vi "phase_two.vi"() -> ()   [LabVIEW 2015]
uses:
  <vilib>/NXT/Block Support/NXT_OutputPort.ctl
  <vilib>/NXT/Block Support/NXT_InputPort.ctl
  <vilib>/NXT/NXTIO Xnodes/NXTIONodeSubVIs/NXTMotorRunDistance.vi
  <vilib>/NXT/Dual Mode Library/Sensors/EV3_Touch_Reset.vi
  <vilib>/NXT/Dual Mode Library/Sound/Tone.vi
  <vilib>/NXT/Dual Mode Library/Waits/Wait_Num.vi
  <vilib>/NXT/Dual Mode Library/Sensors/Touch_Pressed.vi
  <vilib>/NXT/Dual Mode Library/Waits/Wait_Touch.vi
  <vilib>/NXT/Dual Mode Library/Sensors/EV3_Color_RGB.vi
  global1.vi
  all_done?.vi
  <vilib>/NXT/Subs/LVHSConnector.ctl
  <vilib>/NXT/NXTIO Xnodes/AddressXNode/NXTIOAddress.xnode
  <vilib>/NXT/NXTIO Xnodes/NXTIOXNode/NXTIO.xnode
  <vilib>/NXT/LegoClasses/BrickReference/BrickReference.lvclass
panel:
  in  "Slot 8: Small":dbl=69.0
  in  "Slot 8: Big":dbl=64.0
  in  "Slot 7: Small":dbl=61.0
  in  "Slot 7: Big":dbl=58.0
  in  "Slot 6: Small":dbl=54.0
  in  "Slot 6: Big":dbl=54.0
  in  "Slot 5: Small":dbl=46.0
  in  "Slot 5: Big":dbl=46.0
  in  "Slot 4: Small":dbl=38.0
  in  "Slot 4: Big":dbl=38.0
  in  "Slot 3: Small":dbl=30.0
  in  "Slot 3: Big":dbl=30.0
  in  "Slot 2: Small":dbl=22.0
  in  "Slot 2: Big 3":dbl=22.0
  in  "Slot 1: Small":dbl=16.0
  in  "Slot 1: Big":u32=15
  out "Slot 8: Small":bool
  out "Slot 5: Small":bool
  out "Slot 4: Small":bool
  out "Slot 7: Small":bool
  out "Slot 6: Small":bool
  out "Slot 3: Small":bool
  out "Slot 2: Small":bool
  out "Slot 1: Small":bool
  out "Slot 8: Big":bool
  out "Slot 3: Big":bool
  out "Slot 6: Big":bool
  out "Slot 5: Big":bool
  out "Slot 4: Big":bool
  out "Slot 7: Big":bool
  out "Slot 2: Big":bool
  out "Slot 1: Big":bool
  out "Sum Left":i32
  out "ALL DONE?":bool
  out "Trash/Want Case #":u32
  out "Trash?":bool
  out "4: Type 2 #":u8
  out "3: Type 2 #":u8
  out "2: Type 2 #":u8
  out "1: Type 2 #":u8
  out "4: Type 1 #":u8
  out "3: Type 1 #":u8
  out "2: Type 1 #":u8
  out "1: Type 1 #":u8
  out "4: Compound 2":string
  out "4: Compound 1":string
  out "3: Compound 2":string
  out "3: Compound 1":string
  out "2: Compound 2":string
  out "2: Compound 1":string
  out "1: Compound 2":string
  out "1: Compound 1":string
  out "Full?":bool
  out "Stop?":bool
  out "Current Compound":string
  out "Boolean":bool[](array[boolean])
  in  "B Lower 16":u8
  in  "B Upper 16":u8
  in  "G Lower 16":u8
  in  "G Upper 16":u8
  in  "R Lower 16":u8
  in  "R Upper 16":u8
  in  "B Lower 15":u8
  in  "B Upper 15":u8
  in  "G Lower 15":u8
  in  "G Upper 15":u8
  in  "R Lower 15":u8
  in  "R Upper 15":u8
  in  "B Lower 14":u8
  in  "B Upper 14":u8
  in  "G Lower 14":u8
  in  "G Upper 14":u8
  in  "R Lower 14":u8
  in  "R Upper 14":u8
  in  "B Lower 13":u8
  in  "B Upper 13":u8
  in  "G Lower 13":u8
  in  "G Upper 13":u8
  in  "R Lower 13":u8
  in  "R Upper 13":u8
  in  "B Lower 12":u8=5
  in  "B Upper 12":u8=15
  in  "G Lower 12":u8=77
  in  "G Upper 12":u8=90
  in  "R Lower 12":u8=100
  in  "R Upper 12":u8=130
  in  "B Lower 11":u8=18
  in  "B Upper 11":u8=30
  in  "G Lower 11":u8=120
  in  "G Upper 11":u8=150
  in  "R Lower 11":u8=230
  in  "R Upper 11":u8=255
  in  "B Lower 10":u8=10
  in  "B Upper 10":u8=25
  in  "G Lower 10":u8=10
  in  "G Upper 10":u8=20
  in  "R Lower 10":u8=5
  in  "R Upper 10":u8=15
  in  "B Lower 9":u8=55
  in  "B Upper 9":u8=70
  in  "G Lower 9":u8=20
  in  "G Upper 9":u8=35
  in  "R Lower 9":u8=10
  in  "R Upper 9":u8=20
  out "Bool Number":u32
  in  "B Lower 8":u8=5
  in  "B Upper 8":u8=15
  in  "G Lower 8":u8=15
  in  "G Upper 8":u8=25
  in  "R Lower 8":u8=15
  in  "R Upper 8":u8=30
  in  "B Lower 7":u8=16
  in  "B Upper 7":u8=34
  in  "G Lower 7":u8=40
  in  "G Upper 7":u8=66
  in  "R Lower 7":u8=30
  in  "R Upper 7":u8=55
  in  "B Lower 6":u8=50
  in  "B Upper 6":u8=28
  in  "G Lower 6":u8=66
  in  "G Upper 6":u8=96
  in  "R Lower 6":u8=60
  in  "R Upper 6":u8=87
  in  "B Lower 5":u8=86
  in  "B Upper 5":u16=140
  in  "G Lower 5":u8=130
  in  "G Upper 5":u16=170
  in  "R Lower 5":u16=160
  in  "R Upper 5":u16=220
  in  "B Lower 4":u8=7
  in  "B Upper 4":u8=15
  in  "G Lower 4":u8=7
  in  "G Upper 4":u8=11
  in  "R Lower 4":u8=5
  in  "R Upper 4":u8=10
  in  "B Lower 3":u8=45
  in  "B Upper 3":u8=65
  in  "G Lower 3":u8=20
  in  "G Upper 3":u8=45
  in  "R Lower 3":u8=20
  in  "R Upper 3":u8=40
  in  "B Lower 2":u8
  in  "B Upper 2":u8=5
  in  "G Lower 2":u8
  in  "G Upper 2":u8=10
  in  "R Lower 2":u8=30
  in  "R Upper 2":u8=50
  out "What Type?":string
  in  "Cur B":u8=45
  in  "Cur G":u8=75
  in  "\"Cur\" R":u8=70
  out "What Color?":string
  in  "B Lower":u8
  in  "B Upper":u8=10
  in  "G Lower":u8=2
  in  "G Upper":u8=15
  in  "R Upper":u16=110
  in  "R Lower":u8=60
  out "Cur Blue":u8
  out "Cur Green":u8
  out "Cur Red":u8
  out "Current":cluster{"Red":u8, "Green":u8, "Blue":u8}
  # "DEGREES (ENTER POSITIVE NUMBERS)"
  # "REMEMBER BIG NUMBERS ON TOP, SMALL NUMBERS ON BOTTOM"
  # "Red Big"
  # "Red Small"
  # "Blue Big"
  # "Blue Small"
  # "What is needed?"
  # "Possible errors: \nALSO CURRENTLY IN CONTROL MODE\nNOT IN ACTUAL READ COLOR SENSOR MODE\nFOR TESTING PURPOSES*************\n \nwait/time funcitons in loops\n\nNOT ENOUGH SPACE TO SORT? ELONGATE\nDECIDER!!!!!!!"
  # "White Big"
  # "White Small"
  # "HDPE"
  # "Steel"
  # "1) MOTORS: \nA = Top gate\nB = Bottom gate\nC = Scythe\nD = Decider\n\n2) PORTS:\n1) Color\n2) Touch"
  # "Dark Blue Small"
  # "Yellow Small"
  # "Dark Blue Big"
  # "Yellow Big"
  # "Dark Green Big"
  # "Dark Green Small"
  # "Green Big"
  # "Green Small"
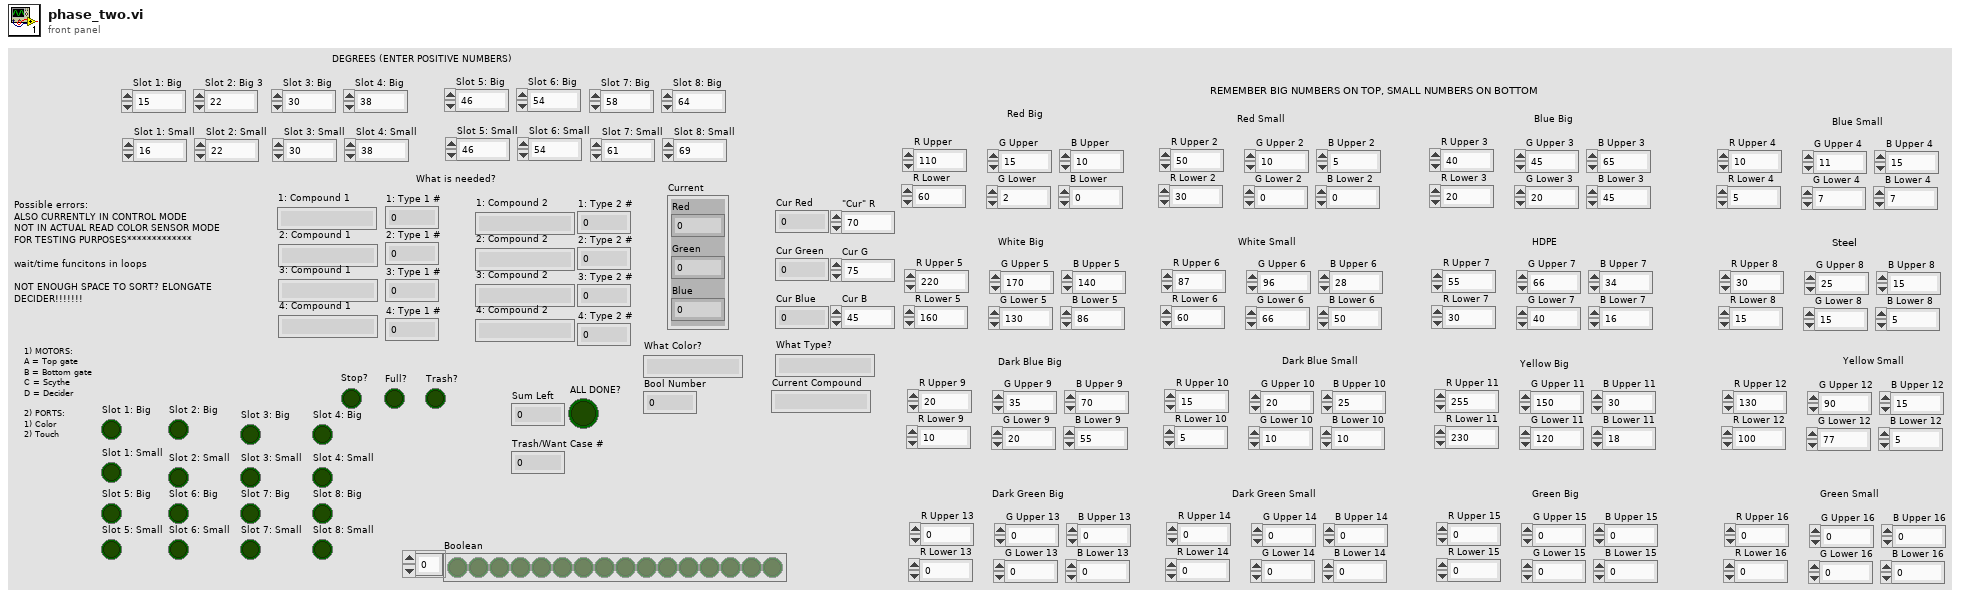
[diagram p1: front panel]
types:
  T1 = typedef "NXT_OutputPort.ctl" = u8
  T2 = typedef "LVHSConnector.ctl" = refnum<class "BrickReference.lvclass">
  T3 = typedef "NXT_InputPort.ctl" = u32
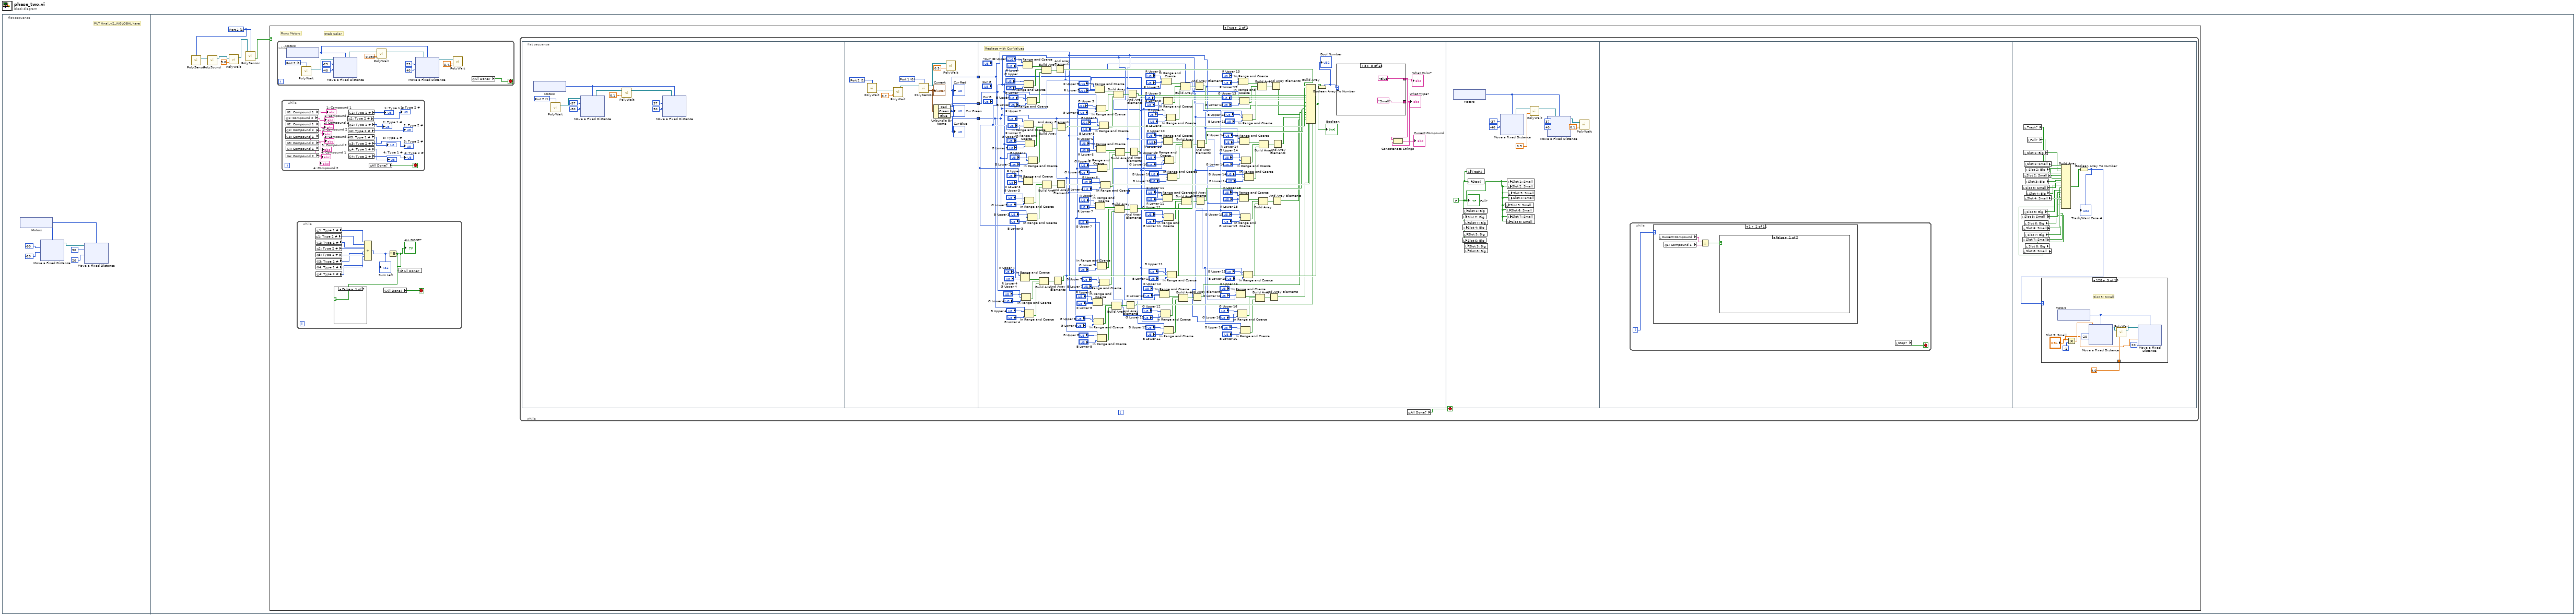
[diagram p0: block diagram]
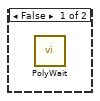
[diagram p2: hidden frame]
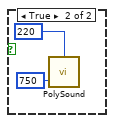
[diagram p3: hidden frame]
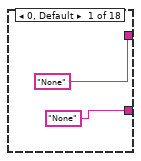
[diagram p4: hidden frame]
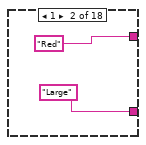
[diagram p5: hidden frame]
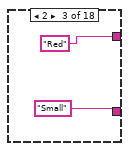
[diagram p6: hidden frame]
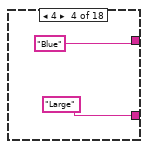
[diagram p7: hidden frame]
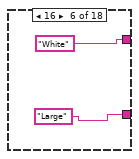
[diagram p8: hidden frame]
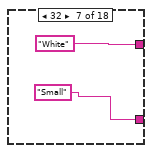
[diagram p9: hidden frame]
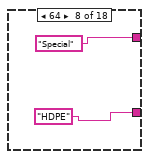
[diagram p10: hidden frame]
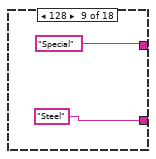
[diagram p11: hidden frame]
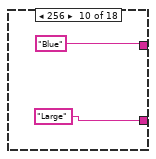
[diagram p12: hidden frame]
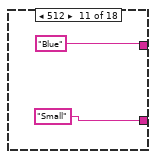
[diagram p13: hidden frame]
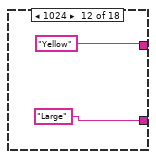
[diagram p14: hidden frame]
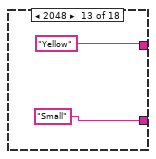
[diagram p15: hidden frame]
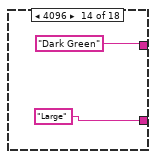
[diagram p16: hidden frame]
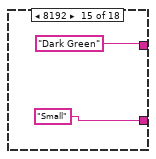
[diagram p17: hidden frame]
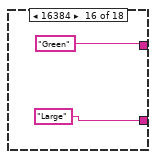
[diagram p18: hidden frame]
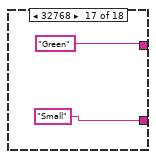
[diagram p19: hidden frame]
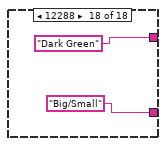
[diagram p20: hidden frame]
diagram:
  n1 = flat-sequence {
    frame #0 {
      # "PUT final_v2_WGLOBAL here"
      n2 = xnode "Motors"() -> ("Motor"=w6:T1)
      n3 = xnode "Move a Fixed Distance"("Speed 1"=-20, "Distance 1"=-90, "Motors"=w6) -> ("NXT/EV3"=w5:T2)  [unwired: 1 in]
      n4 = xnode "Move a Fixed Distance"("Speed 1"=20, "Distance 1"=90, "Motors"=w6, "NXT/EV3"=w5) -> ()  [unwired: 1 out]
    }
    frame #1 {
      w28 = T3 1 items=["Port 1", "Port 2", "Port 3", "Port 4"] ("Port (Port 1)")
      n5 = call-poly <vilib>:"PolySensor.vi"("Port (Port 1)"=w28) -> ("NXT/EV3"=w32:T2)  [unwired: 3 in]
      n6 = call-poly <vilib>:"PolySound.vi"("NXT/EV3"=w32) -> ("NXT/EV3"=w31:T2)  [unwired: 3 in]
      n7 = call-poly <vilib>:"PolyWait.vi"("Time (1 sec)"=sgl 5.0, "NXT/EV3"=w31) -> ("NXT/EV3"=w30:T2)  [unwired: 2 in]
      n8 = call-poly <vilib>:"PolySensor.vi"("NXT/EV3"=w30, "Port (Port 1)"=w28) -> ("Yes / No"=w33:bool)  [unwired: 1 in, 1 out]
      n9 = case shown="True" w33 {
        frame False {
          n10 = call-poly <vilib>:"PolyWait.vi"() -> ()  [unwired: 4 in, 1 out]
        }
        frame True {
          # "Grab Color"
          # "Runs Motors"
          n11 = while {
            stop <- w37 stop-if-true
            w39 = T3 1 items=["Port 1", "Port 2", "Port 3", "Port 4"] ("Port (Port 1)")
            n12 = xnode "Motors"() -> ("Motor"=w45:T1)
            n13 = call-poly <vilib>:"PolyWait.vi"("Port (Port 1)"=w39) -> ("NXT/EV3"=w38:T2)  [unwired: 3 in]
            n14 = xnode "Move a Fixed Distance"("Speed 1"=i8 -40, "Distance 1"=-25, "Motors"=w45, "NXT/EV3"=w38) -> ("NXT/EV3"=w44:T2)
            n15 = call-poly <vilib>:"PolyWait.vi"("Time (1 sec)"=sgl 0.05, "NXT/EV3"=w44) -> ("NXT/EV3"=w43:T2)  [unwired: 2 in]
            n16 = xnode "Move a Fixed Distance"("Speed 1"=i8 40, "Distance 1"=25, "Motors"=w45, "NXT/EV3"=w43) -> ("NXT/EV3"=w34:T2)
            n17 = call-poly <vilib>:"PolyWait.vi"("Time (1 sec)"=sgl 0.4, "NXT/EV3"=w34) -> ()  [unwired: 2 in, 1 out]
            n18 = global read "all_done?.vi" "All Done?"() -> (w37:bool)
          }
          n19 = while {
            stop <- w81 stop-if-true
            n20 = global read "global1.vi" "1: Compound 2"() -> (→"1: Compound 2":string)
            n21 = global read "global1.vi" "2: Compound 2"() -> (→"2: Compound 2":string)
            n22 = global read "global1.vi" "3: Compound 1"() -> (→"3: Compound 1":string)
            n23 = global read "global1.vi" "1: Compound 1"() -> (→"1: Compound 1":string)
            n24 = global read "global1.vi" "2: Compound 1"() -> (→"2: Compound 1":string)
            n25 = global read "global1.vi" "3: Compound 2"() -> (→"3: Compound 2":string)
            n26 = global read "global1.vi" "4: Compound 1"() -> (→"4: Compound 1":string)
            n27 = global read "global1.vi" "4: Compound 2"() -> (→"4: Compound 2":string)
            n28 = global read "global1.vi" "1: Type 2 #"() -> (→"1: Type 2 #":i32)
            n29 = global read "global1.vi" "2: Type 2 #"() -> (→"2: Type 2 #":i32)
            n30 = global read "global1.vi" "3: Type 1 #"() -> (→"3: Type 1 #":i32)
            n31 = global read "global1.vi" "1: Type 1 #"() -> (→"1: Type 1 #":i32)
            n32 = global read "global1.vi" "2: Type 1 #"() -> (→"2: Type 1 #":i32)
            n33 = global read "global1.vi" "3: Type 2 #"() -> (→"3: Type 2 #":i32)
            n34 = global read "global1.vi" "4: Type 1 #"() -> (→"4: Type 1 #":i32)
            n35 = global read "global1.vi" "4: Type 2 #"() -> (→"4: Type 2 #":i32)
            n36 = global read "all_done?.vi" "All Done?"() -> (w81:bool)
          }
          n37 = while {
            stop <- w70 stop-if-true
            n38 = global read "global1.vi" "1: Type 2 #"() -> (w77:i32)
            n39 = global read "global1.vi" "2: Type 2 #"() -> (w75:i32)
            n40 = global read "global1.vi" "3: Type 1 #"() -> (w74:i32)
            n41 = global read "global1.vi" "1: Type 1 #"() -> (w78:i32)
            n42 = global read "global1.vi" "2: Type 1 #"() -> (w76:i32)
            n43 = global read "global1.vi" "3: Type 2 #"() -> (w73:i32)
            n44 = global read "global1.vi" "4: Type 1 #"() -> (w72:i32)
            n45 = global read "global1.vi" "4: Type 2 #"() -> (w71:i32)
            n46 = Compound Arithmetic op=ADD(w78, w77, w76, w75, w74, w73, w72, w71) -> (w69:i32)
            "Sum Left" <- w69
            n47 = global read "all_done?.vi" "All Done?"() -> (w70:bool)
            n48 = Equal To 0?(x=w69) -> (x = 0?=w68:bool)
            "ALL DONE?" <- w68
            n49 = case shown="False" w68 {
              frame False {
              }
              frame True {
                n50 = call-poly <vilib>:"PolySound.vi"("Duration (500 ms)"=u16 750, "Tone (440 Hz)"=u16 220) -> ()  [unwired: 2 in, 1 out]
              }
            }
            n51 = global write "all_done?.vi" "All Done?"(w68) -> ()
          }
          n52 = while {
            stop <- w101 stop-if-true
            n53 = flat-sequence {
              tunnel: [w135] -> w100
              tunnel: [w134] -> w99
              tunnel: [w133] -> w98
              tunnel: w100 -> [w146]
              tunnel: w99 -> [w145]
              tunnel: w98 -> [w144]
              frame #0 {
                w103 = T3 1 items=["Port 1", "Port 2", "Port 3", "Port 4"] ("Port (Port 1)")
                n54 = xnode "Motors"() -> ("Motor"=w110:T1)
                n55 = call-poly <vilib>:"PolyWait.vi"("Port (Port 1)"=w103) -> ("NXT/EV3"=w102:T2)  [unwired: 3 in]
                n56 = xnode "Move a Fixed Distance"("Speed 1"=i8 -50, "Distance 1"=-37, "Motors"=w110, "NXT/EV3"=w102) -> ("NXT/EV3"=w109:T2)
                n57 = call-poly <vilib>:"PolyWait.vi"("Time (1 sec)"=0.1, "NXT/EV3"=w109) -> ("NXT/EV3"=w108:T2)  [unwired: 2 in]
                n58 = xnode "Move a Fixed Distance"("Speed 1"=i8 50, "Distance 1"=37, "Motors"=w110, "NXT/EV3"=w108) -> ()  [unwired: 1 out]
              }
              frame #1 {
                w139 = T3 0 items=["Port 1", "Port 2", "Port 3", "Port 4"] ("Port (Port 1)")
                w142 = T3 1 items=["Port 1", "Port 2", "Port 3", "Port 4"] ("Port (Port 1)")
                n59 = call-poly <vilib>:"PolyWait.vi"("Port (Port 1)"=w142) -> ("NXT/EV3"=w141:T2)  [unwired: 3 in]
                n60 = call-poly <vilib>:"PolyWait.vi"("Time (1 sec)"=0.7, "NXT/EV3"=w141) -> ("NXT/EV3"=w140:T2)  [unwired: 2 in]
                n61 = call-poly <vilib>:"PolySensor.vi"("NXT/EV3"=w140, "Port (Port 1)"=w139) -> ("RGB Color"=w138:cluster{"Red":u8, "Green":u8, "Blue":u8}, "NXT/EV3"=w137:T2)  [unwired: 1 in]
                "Current" <- w138
                n62 = Unbundle By Name(w138) -> ("Red"=w135:u8, "Green"=w134:u8, "Blue"=w133:u8)
                "Cur Green" <- w134
                "Cur Red" <- w135
                "Cur Blue" <- w133
                n63 = call-poly <vilib>:"PolyWait.vi"("Time (1 sec)"=sgl 0.5, "NXT/EV3"=w137) -> ()  [unwired: 2 in, 1 out]
              }
              frame #2 {
                # "Replace with Cur Values"
                n64 = In Range and Coerce(upper limit="R Upper 4", x=w146, lower limit="R Lower 4") -> (In Range?=w288:bool)  [unwired: 1 out]
                n65 = In Range and Coerce(upper limit="G Upper 4", x=w145, lower limit="G Lower 4") -> (In Range?=w287:bool)  [unwired: 1 out]
                n66 = In Range and Coerce(upper limit="R Upper", x=w146, lower limit="R Lower") -> (In Range?=w321:bool)  [unwired: 1 out]
                n67 = In Range and Coerce(upper limit="R Upper 3", x=w146, lower limit="R Lower 3") -> (In Range?=w298:bool)  [unwired: 1 out]
                n68 = In Range and Coerce(upper limit="G Upper", x=w145, lower limit="G Lower") -> (In Range?=w320:bool)  [unwired: 1 out]
                n69 = In Range and Coerce(upper limit="R Upper 2", x=w146, lower limit="R Lower 2") -> (In Range?=w310:bool)  [unwired: 1 out]
                n70 = In Range and Coerce(upper limit="G Upper 3", x=w145, lower limit="G Lower 3") -> (In Range?=w297:bool)  [unwired: 1 out]
                n71 = In Range and Coerce(upper limit="B Upper 4", x=w144, lower limit="B Lower 4") -> (In Range?=w285:bool)  [unwired: 1 out]
                n72 = In Range and Coerce(upper limit="G Upper 2", x=w145, lower limit="G Lower 2") -> (In Range?=w309:bool)  [unwired: 1 out]
                n73 = In Range and Coerce(upper limit="B Upper", x=w144, lower limit="B Lower") -> (In Range?=w306:bool)  [unwired: 1 out]
                n74 = In Range and Coerce(upper limit="B Upper 3", x=w144, lower limit="B Lower 3") -> (In Range?=w295:bool)  [unwired: 1 out]
                n75 = In Range and Coerce(upper limit="B Upper 2", x=w144, lower limit="B Lower 2") -> (In Range?=w305:bool)  [unwired: 1 out]
                n76 = Build Array(w288, w287, w285) -> (w286:bool[])
                n77 = Build Array(w321, w320, w306) -> (w319:bool[])
                n78 = Build Array(w298, w297, w295) -> (w296:bool[])
                n79 = Build Array(w310, w309, w305) -> (w308:bool[])
                n80 = And Array Elements(Boolean array=w286) -> (logical AND=w284:bool)
                n81 = And Array Elements(Boolean array=w319) -> (logical AND=w318:bool)
                n82 = And Array Elements(Boolean array=w296) -> (logical AND=w283:bool)
                n83 = And Array Elements(Boolean array=w308) -> (logical AND=w307:bool)
                n84 = In Range and Coerce(upper limit="R Upper 8", x=w146, lower limit="R Lower 8") -> (In Range?=w246:bool)  [unwired: 1 out]
                n85 = In Range and Coerce(upper limit="G Upper 8", x=w145, lower limit="G Lower 8") -> (In Range?=w245:bool)  [unwired: 1 out]
                n86 = In Range and Coerce(upper limit="R Upper 5", x=w146, lower limit="R Lower 5") -> (In Range?=w276:bool)  [unwired: 1 out]
                n87 = In Range and Coerce(upper limit="R Upper 7", x=w146, lower limit="R Lower 7") -> (In Range?=w256:bool)  [unwired: 1 out]
                n88 = In Range and Coerce(upper limit="G Upper 5", x=w145, lower limit="G Lower 5") -> (In Range?=w275:bool)  [unwired: 1 out]
                n89 = In Range and Coerce(upper limit="R Upper 6", x=w146, lower limit="R Lower 6") -> (In Range?=w267:bool)  [unwired: 1 out]
                n90 = In Range and Coerce(upper limit="G Upper 7", x=w145, lower limit="G Lower 7") -> (In Range?=w255:bool)  [unwired: 1 out]
                n91 = In Range and Coerce(upper limit="B Upper 8", x=w144, lower limit="B Lower 8") -> (In Range?=w243:bool)  [unwired: 1 out]
                n92 = In Range and Coerce(upper limit="G Upper 6", x=w145, lower limit="G Lower 6") -> (In Range?=w266:bool)  [unwired: 1 out]
                n93 = In Range and Coerce(upper limit="B Upper 5", x=w144, lower limit="B Lower 5") -> (In Range?=w264:bool)  [unwired: 1 out]
                n94 = In Range and Coerce(upper limit="B Upper 7", x=w144, lower limit="B Lower 7") -> (In Range?=w253:bool)  [unwired: 1 out]
                n95 = In Range and Coerce(upper limit="B Upper 6", x=w144, lower limit="B Lower 6") -> (In Range?=w263:bool)  [unwired: 1 out]
                n96 = Build Array(w246, w245, w243) -> (w244:bool[])
                n97 = Build Array(w276, w275, w264) -> (w274:bool[])
                n98 = Build Array(w256, w255, w253) -> (w254:bool[])
                n99 = Build Array(w267, w266, w263) -> (w265:bool[])
                n100 = And Array Elements(Boolean array=w244) -> (logical AND=w239:bool)
                n101 = And Array Elements(Boolean array=w274) -> (logical AND=w242:bool)
                n102 = And Array Elements(Boolean array=w254) -> (logical AND=w240:bool)
                n103 = And Array Elements(Boolean array=w265) -> (logical AND=w241:bool)
                n104 = In Range and Coerce(upper limit="R Upper 12", x=w146, lower limit="R Lower 12") -> (In Range?=w201:bool)  [unwired: 1 out]
                n105 = In Range and Coerce(upper limit="G Upper 12", x=w145, lower limit="G Lower 12") -> (In Range?=w200:bool)  [unwired: 1 out]
                n106 = In Range and Coerce(upper limit="R Upper 9", x=w146, lower limit="R Lower 9") -> (In Range?=w231:bool)  [unwired: 1 out]
                n107 = In Range and Coerce(upper limit="R Upper 11", x=w146, lower limit="R Lower 11") -> (In Range?=w211:bool)  [unwired: 1 out]
                n108 = In Range and Coerce(upper limit="G Upper 9", x=w145, lower limit="G Lower 9") -> (In Range?=w230:bool)  [unwired: 1 out]
                n109 = In Range and Coerce(upper limit="R Upper 10", x=w146, lower limit="R Lower 10") -> (In Range?=w222:bool)  [unwired: 1 out]
                n110 = In Range and Coerce(upper limit="G Upper 11", x=w145, lower limit="G Lower 11") -> (In Range?=w210:bool)  [unwired: 1 out]
                n111 = In Range and Coerce(upper limit="B Upper 12", x=w144, lower limit="B Lower 12") -> (In Range?=w198:bool)  [unwired: 1 out]
                n112 = In Range and Coerce(upper limit="G Upper 10", x=w145, lower limit="G Lower 10") -> (In Range?=w221:bool)  [unwired: 1 out]
                n113 = In Range and Coerce(upper limit="B Upper 9", x=w144, lower limit="B Lower 9") -> (In Range?=w219:bool)  [unwired: 1 out]
                n114 = In Range and Coerce(upper limit="B Upper 11", x=w144, lower limit="B Lower 11") -> (In Range?=w208:bool)  [unwired: 1 out]
                n115 = In Range and Coerce(upper limit="B Upper 10", x=w144, lower limit="B Lower 10") -> (In Range?=w218:bool)  [unwired: 1 out]
                n116 = Build Array(w201, w200, w198) -> (w199:bool[])
                n117 = Build Array(w231, w230, w219) -> (w229:bool[])
                n118 = Build Array(w211, w210, w208) -> (w209:bool[])
                n119 = Build Array(w222, w221, w218) -> (w220:bool[])
                n120 = And Array Elements(Boolean array=w199) -> (logical AND=w154:bool)
                n121 = And Array Elements(Boolean array=w229) -> (logical AND=w157:bool)
                n122 = And Array Elements(Boolean array=w209) -> (logical AND=w155:bool)
                n123 = And Array Elements(Boolean array=w220) -> (logical AND=w156:bool)
                n124 = In Range and Coerce(upper limit="R Upper 16", x=w146, lower limit="R Lower 16") -> (In Range?=w161:bool)  [unwired: 1 out]
                n125 = In Range and Coerce(upper limit="G Upper 16", x=w145, lower limit="G Lower 16") -> (In Range?=w160:bool)  [unwired: 1 out]
                n126 = In Range and Coerce(upper limit="R Upper 13", x=w146, lower limit="R Lower 13") -> (In Range?=w191:bool)  [unwired: 1 out]
                n127 = In Range and Coerce(upper limit="R Upper 15", x=w146, lower limit="R Lower 15") -> (In Range?=w171:bool)  [unwired: 1 out]
                n128 = In Range and Coerce(upper limit="G Upper 13", x=w145, lower limit="G Lower 13") -> (In Range?=w190:bool)  [unwired: 1 out]
                n129 = In Range and Coerce(upper limit="R Upper 14", x=w146, lower limit="R Lower 14") -> (In Range?=w182:bool)  [unwired: 1 out]
                n130 = In Range and Coerce(upper limit="G Upper 15", x=w145, lower limit="G Lower 15") -> (In Range?=w170:bool)  [unwired: 1 out]
                n131 = In Range and Coerce(upper limit="B Upper 16", x=w144, lower limit="B Lower 16") -> (In Range?=w158:bool)  [unwired: 1 out]
                n132 = In Range and Coerce(upper limit="G Upper 14", x=w145, lower limit="G Lower 14") -> (In Range?=w181:bool)  [unwired: 1 out]
                n133 = In Range and Coerce(upper limit="B Upper 13", x=w144, lower limit="B Lower 13") -> (In Range?=w179:bool)  [unwired: 1 out]
                n134 = In Range and Coerce(upper limit="B Upper 15", x=w144, lower limit="B Lower 15") -> (In Range?=w168:bool)  [unwired: 1 out]
                n135 = In Range and Coerce(upper limit="B Upper 14", x=w144, lower limit="B Lower 14") -> (In Range?=w178:bool)  [unwired: 1 out]
                n136 = Build Array(w161, w160, w158) -> (w159:bool[])
                n137 = Build Array(w191, w190, w179) -> (w189:bool[])
                n138 = Build Array(w171, w170, w168) -> (w169:bool[])
                n139 = Build Array(w182, w181, w178) -> (w180:bool[])
                n140 = And Array Elements(Boolean array=w159) -> (logical AND=w150:bool)
                n141 = And Array Elements(Boolean array=w189) -> (logical AND=w153:bool)
                n142 = And Array Elements(Boolean array=w169) -> (logical AND=w151:bool)
                n143 = And Array Elements(Boolean array=w180) -> (logical AND=w152:bool)
                n144 = Build Array(w318, w307, w283, w284, w242, w241, w240, w239, w157, w156, w155, w154, w153, w152, w151, w150) -> (w317:bool[])
                "Boolean" <- w317
                n145 = Boolean Array To Number(Boolean array=w317) -> (number=w238:u32)
                "Bool Number" <- w238
                n146 = case shown="8" w238 {
                  tunnel: ["None" "Red" "Red" "Blue" "Blue" "White" "White" "Special" "Special" "Blue" "Blue" "Yellow" "Yellow" "Dark Green" "Dark Green" "Green" "Green" "Dark Green"] -> w149
                  tunnel: ["None" "Large" "Small" "Large" "Small" "Large" "Small" "HDPE" "Steel" "Large" "Small" "Large" "Small" "Large" "Small" "Large" "Small" "Big/Small"] -> w148
                  frame 0, Default {
                  }
                  frame 1 {
                  }
                  frame 2 {
                  }
                  frame 4 {
                  }
                  frame 8 {
                  }
                  frame 16 {
                  }
                  frame 32 {
                  }
                  frame 64 {
                  }
                  frame 128 {
                  }
                  frame 256 {
                  }
                  frame 512 {
                  }
                  frame 1024 {
                  }
                  frame 2048 {
                  }
                  frame 4096 {
                  }
                  frame 8192 {
                  }
                  frame 16384 {
                  }
                  frame 32768 {
                  }
                  frame 12288 {
                  }
                }
                "What Color?" <- w149
                "What Type?" <- w148
                n147 = Concatenate Strings(w149, w148) -> (→"Current Compound":string)
              }
              frame #3 {
                w366 = FALSE
                n148 = xnode "Motors"() -> ("Motor"=w372:T1)
                n149 = local write "Slot 2: Big"(w366) -> ()
                n150 = local write "Slot 6: Big"(w366) -> ()
                n151 = local write "Slot 4: Big"(w366) -> ()
                n152 = local write "Slot 1: Big"(w366) -> ()
                n153 = local write "Slot 5: Big"(w366) -> ()
                n154 = local write "Slot 7: Big"(w366) -> ()
                n155 = local write "Slot 3: Big"(w366) -> ()
                n156 = local write "Slot 8: Big"(w366) -> ()
                n157 = local write "Trash?"(w366) -> ()
                n158 = local write "Stop?"(w366) -> ()
                n159 = xnode "Move a Fixed Distance"("Speed 1"=i8 -40 ("Power/Speed 1"), "Distance 1"=-37, "Motors"=w372) -> ("NXT/EV3"=w374:T2)  [unwired: 1 in]
                n160 = local write "Slot 5: Small"(w366) -> ()
                n161 = local write "Slot 6: Small"(w366) -> ()
                n162 = local write "Slot 8: Small"(w366) -> ()
                n163 = local write "Slot 1: Small"(w366) -> ()
                n164 = local write "Slot 2: Small"(w366) -> ()
                n165 = local write "Slot 7: Small"(w366) -> ()
                n166 = local write "Slot 3: Small"(w366) -> ()
                n167 = local write "Slot 4: Small"(w366) -> ()
                n168 = call-poly <vilib>:"PolyWait.vi"("Time (1 sec)"=0.3, "NXT/EV3"=w374) -> ("NXT/EV3"=w373:T2)  [unwired: 2 in]
                n169 = xnode "Move a Fixed Distance"("Speed 1"=i8 40, "Distance 1"=37, "Motors"=w372, "NXT/EV3"=w373) -> ("NXT/EV3"=w364:T2)
                n170 = call-poly <vilib>:"PolyWait.vi"("Time (1 sec)"=sgl 0.1, "NXT/EV3"=w364) -> ()  [unwired: 2 in, 1 out]
                "Full?" <- w366
              }
              frame #4 {
                n171 = while {
                  i -> [w396]
                  stop <- w397 stop-if-true
                  n172 = case shown="1" w396 {
                    frame 0, Default {
                    }
                    frame 1 {
                      n173 = local read "Current Compound"() -> (w400:string)
                      n174 = global read "global1.vi" "1: Compound 1"() -> (w399:string)
                      n175 = Equal?(x=w400, y=w399) -> (x = y?=w398:bool)
                      n176 = case shown="False" w398 {
                        frame False {
                        }
                        frame True {
                          n177 = global read "global1.vi" "1: Type 1 #"() -> (w402:i32)
                          n178 = Greater?(x=w402, y=u32 0) -> (0:w401:bool)
                          n179 = case shown="False" w401 {
                            frame False {
                              n180 = local write "Stop?"(TRUE) -> ()
                              "Slot 5: Big" <- TRUE
                            }
                            frame True {
                              n181 = global read "global1.vi" "1: Type 1 #"() -> (w409:i32)
                              n182 = Decrement(x=w409) -> (x-1=w408:i32)
                              n183 = global write "global1.vi" "1: Type 1 #"(w408) -> ()
                              "Stop?" <- TRUE
                              "Slot 1: Big" <- TRUE
                            }
                          }
                        }
                      }
                    }
                    frame 2 {
                      n184 = local read "Current Compound"() -> (w412:string)
                      n185 = global read "global1.vi" "1: Compound 2"() -> (w411:string)
                      n186 = Equal?(x=w412, y=w411) -> (x = y?=w410:bool)
                      n187 = case shown="True" w410 {
                        frame False {
                        }
                        frame True {
                          n188 = global read "global1.vi" "1: Type 2 #"() -> (w414:i32)
                          n189 = Greater?(x=w414, y=u32 0) -> (0:w413:bool)
                          n190 = case shown="False" w413 {
                            frame False {
                              n191 = local write "Stop?"(TRUE) -> ()
                              "Slot 5: Small" <- TRUE
                            }
                            frame True {
                              n192 = global read "global1.vi" "1: Type 2 #"() -> (w421:i32)
                              n193 = local write "Stop?"(TRUE) -> ()
                              n194 = Decrement(x=w421) -> (x-1=w420:i32)
                              n195 = global write "global1.vi" "1: Type 2 #"(w420) -> ()
                              "Slot 1: Small" <- TRUE
                            }
                          }
                        }
                      }
                    }
                    frame 3 {
                      n196 = local read "Current Compound"() -> (w424:string)
                      n197 = global read "global1.vi" "2: Compound 1"() -> (w423:string)
                      n198 = Equal?(x=w424, y=w423) -> (x = y?=w422:bool)
                      n199 = case shown="True" w422 {
                        frame False {
                        }
                        frame True {
                          n200 = global read "global1.vi" "2: Type 1 #"() -> (w426:i32)
                          n201 = Greater?(x=w426, y=u32 0) -> (0:w425:bool)
                          n202 = case shown="True" w425 {
                            frame False {
                              n203 = local write "Stop?"(TRUE) -> ()
                              "Slot 6: Big" <- TRUE
                            }
                            frame True {
                              n204 = global read "global1.vi" "2: Type 1 #"() -> (w433:i32)
                              n205 = local write "Stop?"(TRUE) -> ()
                              n206 = Decrement(x=w433) -> (x-1=w432:i32)
                              n207 = global write "global1.vi" "2: Type 1 #"(w432) -> ()
                              "Slot 2: Big" <- TRUE
                            }
                          }
                        }
                      }
                    }
                    frame 4 {
                      n208 = local read "Current Compound"() -> (w436:string)
                      n209 = global read "global1.vi" "2: Compound 2"() -> (w435:string)
                      n210 = Equal?(x=w436, y=w435) -> (x = y?=w434:bool)
                      n211 = case shown="True" w434 {
                        frame False {
                        }
                        frame True {
                          n212 = global read "global1.vi" "2: Type 2 #"() -> (w438:i32)
                          n213 = Greater?(x=w438, y=u32 0) -> (0:w437:bool)
                          n214 = case shown="False" w437 {
                            frame False {
                              n215 = local write "Stop?"(TRUE) -> ()
                              "Slot 6: Small" <- TRUE
                            }
                            frame True {
                              n216 = global read "global1.vi" "2: Type 2 #"() -> (w445:i32)
                              n217 = local write "Stop?"(TRUE) -> ()
                              n218 = Decrement(x=w445) -> (x-1=w444:i32)
                              n219 = global write "global1.vi" "2: Type 2 #"(w444) -> ()
                              "Slot 2: Small" <- TRUE
                            }
                          }
                        }
                      }
                    }
                    frame 5 {
                      n220 = local read "Current Compound"() -> (w448:string)
                      n221 = global read "global1.vi" "3: Compound 1"() -> (w447:string)
                      n222 = Equal?(x=w448, y=w447) -> (x = y?=w446:bool)
                      n223 = case shown="True" w446 {
                        frame False {
                        }
                        frame True {
                          n224 = global read "global1.vi" "3: Type 1 #"() -> (w450:i32)
                          n225 = Greater?(x=w450, y=u32 0) -> (0:w449:bool)
                          n226 = case shown="True" w449 {
                            frame False {
                              n227 = local write "Stop?"(TRUE) -> ()
                              "Slot 3: Big" <- TRUE
                            }
                            frame True {
                              n228 = global read "global1.vi" "3: Type 1 #"() -> (w457:i32)
                              n229 = local write "Stop?"(TRUE) -> ()
                              n230 = Decrement(x=w457) -> (x-1=w456:i32)
                              n231 = global write "global1.vi" "3: Type 1 #"(w456) -> ()
                              "Slot 7: Big" <- TRUE
                            }
                          }
                        }
                      }
                    }
                    frame 6 {
                      n232 = local read "Current Compound"() -> (w460:string)
                      n233 = global read "global1.vi" "3: Compound 2"() -> (w459:string)
                      n234 = Equal?(x=w460, y=w459) -> (x = y?=w458:bool)
                      n235 = case shown="True" w458 {
                        frame False {
                        }
                        frame True {
                          n236 = global read "global1.vi" "3: Type 2 #"() -> (w462:i32)
                          n237 = Greater?(x=w462, y=u32 0) -> (0:w461:bool)
                          n238 = case shown="False" w461 {
                            frame False {
                              n239 = local write "Stop?"(TRUE) -> ()
                              "Slot 7: Small" <- TRUE
                            }
                            frame True {
                              n240 = global read "global1.vi" "3: Type 2 #"() -> (w469:i32)
                              n241 = local write "Stop?"(TRUE) -> ()
                              n242 = Decrement(x=w469) -> (x-1=w468:i32)
                              n243 = global write "global1.vi" "3: Type 2 #"(w468) -> ()
                              "Slot 3: Small" <- TRUE
                            }
                          }
                        }
                      }
                    }
                    frame 7 {
                      n244 = local read "Current Compound"() -> (w472:string)
                      n245 = global read "global1.vi" "4: Compound 1"() -> (w471:string)
                      n246 = Equal?(x=w472, y=w471) -> (x = y?=w470:bool)
                      n247 = case shown="True" w470 {
                        frame False {
                        }
                        frame True {
                          n248 = global read "global1.vi" "4: Type 1 #"() -> (w474:i32)
                          n249 = Greater?(x=w474, y=u32 0) -> (0:w473:bool)
                          n250 = case shown="False" w473 {
                            frame False {
                              n251 = local write "Stop?"(TRUE) -> ()
                              "Slot 8: Big" <- TRUE
                            }
                            frame True {
                              n252 = global read "global1.vi" "4: Type 1 #"() -> (w481:i32)
                              n253 = local write "Stop?"(TRUE) -> ()
                              n254 = Decrement(x=w481) -> (x-1=w480:i32)
                              n255 = global write "global1.vi" "4: Type 1 #"(w480) -> ()
                              "Slot 4: Big" <- TRUE
                            }
                          }
                        }
                      }
                    }
                    frame 8 {
                      n256 = local read "Current Compound"() -> (w484:string)
                      n257 = global read "global1.vi" "4: Compound 2"() -> (w483:string)
                      n258 = Equal?(x=w484, y=w483) -> (x = y?=w482:bool)
                      n259 = case shown="True" w482 {
                        frame False {
                        }
                        frame True {
                          n260 = global read "global1.vi" "4: Type 2 #"() -> (w486:i32)
                          n261 = Greater?(x=w486, y=u32 0) -> (0:w485:bool)
                          n262 = case shown="False" w485 {
                            frame False {
                              n263 = local write "Stop?"(TRUE) -> ()
                              "Slot 8: Small" <- TRUE
                            }
                            frame True {
                              n264 = global read "global1.vi" "4: Type 2 #"() -> (w493:i32)
                              n265 = local write "Stop?"(TRUE) -> ()
                              n266 = Decrement(x=w493) -> (x-1=w492:i32)
                              n267 = global write "global1.vi" "4: Type 2 #"(w492) -> ()
                              "Slot 4: Small" <- TRUE
                            }
                          }
                        }
                      }
                    }
                    frame 9 {
                    }
                    frame 10 {
                      w494 = TRUE
                      n268 = local write "Stop?"(w494) -> ()
                      "Trash?" <- w494
                    }
                  }
                  n269 = local read "Stop?"() -> (w397:bool)
                }
              }
              frame #5 {
                n270 = local read "Slot 5: Small"() -> (w501:bool)
                n271 = local read "Slot 3: Small"() -> (w506:bool)
                n272 = local read "Slot 6: Small"() -> (w499:bool)
                n273 = local read "Slot 7: Small"() -> (w497:bool)
                n274 = local read "Slot 8: Small"() -> (w495:bool)
                n275 = local read "Slot 2: Small"() -> (w508:bool)
                n276 = local read "Slot 5: Big"() -> (w502:bool)
                n277 = local read "Trash?"() -> (w515:bool)
                n278 = local read "Slot 1: Big"() -> (w511:bool)
                n279 = local read "Slot 1: Small"() -> (w510:bool)
                n280 = local read "Slot 4: Small"() -> (w504:bool)
                n281 = local read "Slot 6: Big"() -> (w500:bool)
                n282 = local read "Slot 7: Big"() -> (w498:bool)
                n283 = local read "Slot 3: Big"() -> (w507:bool)
                n284 = local read "Slot 2: Big"() -> (w509:bool)
                n285 = local read "Slot 8: Big"() -> (w496:bool)
                n286 = local read "Slot 4: Big"() -> (w505:bool)
                n287 = local read "Full?"() -> (w514:bool)
                n288 = Build Array(w515, w514, w511, w510, w509, w508, w507, w506, w505, w504, w502, w501, w500, w499, w498, w497, w496, w495) -> (w513:bool[])
                n289 = Boolean Array To Number(Boolean array=w513) -> (number=w512:u32)
                "Trash/Want Case #" <- w512
                n290 = case shown="128" w512 {
                  tunnel: sgl 4.0 ("Time (1 sec)") -> [_ w517 w546 w579 w608 w638 w668 w699 w728 w759 w788 w818 w849 w879 w908 w939 w968 w998 w1028]
                  frame 0, Default {
                    # "All Done"
                    n291 = call-poly <vilib>:"PolySound.vi"("Duration (500 ms)"=u16 2000) -> ()  [unwired: 3 in, 1 out]
                  }
                  frame 1 {
                    # "Trash"
                    n292 = xnode "Motors"() -> ("Motor"=w521:T1)
                    n293 = xnode "Move a Fixed Distance"("Speed 1"=i8 -30, "Distance 1"=-90, "Motors"=w521) -> ("NXT/EV3"=w522:T2)  [unwired: 1 in]
                    n294 = call-poly <vilib>:"PolyWait.vi"("Time (1 sec)"=w517, "NXT/EV3"=w522) -> ("NXT/EV3"=w523:T2)  [unwired: 2 in]
                    n295 = xnode "Move a Fixed Distance"("Speed 1"=i8 30, "Distance 1"=90, "Motors"=w521, "NXT/EV3"=w523) -> ()  [unwired: 1 out]
                  }
                  frame 2 {
                    # "Full"
                    n296 = xnode "Motors"() -> ("Motor"=w550:T1)
                    n297 = xnode "Move a Fixed Distance"("Speed 1"=i8 -20, "Distance 1"=-82, "Motors"=w550) -> ("NXT/EV3"=w551:T2)  [unwired: 1 in]
                    n298 = call-poly <vilib>:"PolyWait.vi"("Time (1 sec)"=w546, "NXT/EV3"=w551) -> ("NXT/EV3"=w552:T2)  [unwired: 2 in]
                    n299 = xnode "Move a Fixed Distance"("Speed 1"=i8 20, "Distance 1"=82, "Motors"=w550, "NXT/EV3"=w552) -> ()  [unwired: 1 out]
                  }
                  frame 4 {
                    # "Slot 1: Big"
                    n300 = xnode "Motors"() -> ("Motor"=w581:T1)
                    n301 = Multiply(x="Slot 1: Big", y=-1) -> (x*y=w577:u32)
                    n302 = xnode "Move a Fixed Distance"("Speed 1"=i8 -20, "Distance 1"=w577, "Motors"=w581) -> ("NXT/EV3"=w582:T2)  [unwired: 1 in]
                    n303 = call-poly <vilib>:"PolyWait.vi"("Time (1 sec)"=w579, "NXT/EV3"=w582) -> ("NXT/EV3"=w583:T2)  [unwired: 2 in]
                    n304 = xnode "Move a Fixed Distance"("Speed 1"=i8 20, "Distance 1"="Slot 1: Big", "Motors"=w581, "NXT/EV3"=w583) -> ()  [unwired: 1 out]
                  }
                  frame 8 {
                    # "Slot 1: Small"
                    n305 = xnode "Motors"() -> ("Motor"=w611:T1)
                    n306 = Multiply(x="Slot 1: Small", y=-1) -> (x*y=w606:dbl)
                    n307 = xnode "Move a Fixed Distance"("Speed 1"=i8 -20, "Distance 1"=w606, "Motors"=w611) -> ("NXT/EV3"=w612:T2)  [unwired: 1 in]
                    n308 = call-poly <vilib>:"PolyWait.vi"("Time (1 sec)"=w608, "NXT/EV3"=w612) -> ("NXT/EV3"=w613:T2)  [unwired: 2 in]
                    n309 = xnode "Move a Fixed Distance"("Speed 1"=i8 20, "Distance 1"="Slot 1: Small", "Motors"=w611, "NXT/EV3"=w613) -> ()  [unwired: 1 out]
                  }
                  frame 16 {
                    # "Slot 2: Big"
                    n310 = xnode "Motors"() -> ("Motor"=w641:T1)
                    n311 = Multiply(x="Slot 2: Big 3", y=-1) -> (x*y=w636:dbl)
                    n312 = xnode "Move a Fixed Distance"("Speed 1"=i8 -20, "Distance 1"=w636, "Motors"=w641) -> ("NXT/EV3"=w642:T2)  [unwired: 1 in]
                    n313 = call-poly <vilib>:"PolyWait.vi"("Time (1 sec)"=w638, "NXT/EV3"=w642) -> ("NXT/EV3"=w643:T2)  [unwired: 2 in]
                    n314 = xnode "Move a Fixed Distance"("Speed 1"=i8 20, "Distance 1"="Slot 2: Big 3", "Motors"=w641, "NXT/EV3"=w643) -> ()  [unwired: 1 out]
                  }
                  frame 32 {
                    # "Slot 2: Small"
                    n315 = xnode "Motors"() -> ("Motor"=w671:T1)
                    n316 = Multiply(x="Slot 2: Small", y=-1) -> (x*y=w666:dbl)
                    n317 = xnode "Move a Fixed Distance"("Speed 1"=i8 -20, "Distance 1"=w666, "Motors"=w671) -> ("NXT/EV3"=w672:T2)  [unwired: 1 in]
                    n318 = call-poly <vilib>:"PolyWait.vi"("Time (1 sec)"=w668, "NXT/EV3"=w672) -> ("NXT/EV3"=w673:T2)  [unwired: 2 in]
                    n319 = xnode "Move a Fixed Distance"("Speed 1"=i8 20, "Distance 1"="Slot 2: Small", "Motors"=w671, "NXT/EV3"=w673) -> ()  [unwired: 1 out]
                  }
                  frame 64 {
                    # "Slot 3: Big"
                    n320 = xnode "Motors"() -> ("Motor"=w701:T1)
                    n321 = Multiply(x="Slot 3: Big", y=-1) -> (x*y=w697:dbl)
                    n322 = xnode "Move a Fixed Distance"("Speed 1"=i8 -20, "Distance 1"=w697, "Motors"=w701) -> ("NXT/EV3"=w702:T2)  [unwired: 1 in]
                    n323 = call-poly <vilib>:"PolyWait.vi"("Time (1 sec)"=w699, "NXT/EV3"=w702) -> ("NXT/EV3"=w703:T2)  [unwired: 2 in]
                    n324 = xnode "Move a Fixed Distance"("Speed 1"=i8 20, "Distance 1"="Slot 3: Big", "Motors"=w701, "NXT/EV3"=w703) -> ()  [unwired: 1 out]
                  }
                  frame 128 {
                    # "Slot 3: Small"
                    n325 = xnode "Motors"() -> ("Motor"=w731:T1)
                    n326 = Multiply(x="Slot 3: Small", y=-1) -> (x*y=w726:dbl)
                    n327 = xnode "Move a Fixed Distance"("Speed 1"=i8 -20, "Distance 1"=w726, "Motors"=w731) -> ("NXT/EV3"=w732:T2)  [unwired: 1 in]
                    n328 = call-poly <vilib>:"PolyWait.vi"("Time (1 sec)"=w728, "NXT/EV3"=w732) -> ("NXT/EV3"=w733:T2)  [unwired: 2 in]
                    n329 = xnode "Move a Fixed Distance"("Speed 1"=i8 20, "Distance 1"="Slot 3: Small", "Motors"=w731, "NXT/EV3"=w733) -> ()  [unwired: 1 out]
                  }
                  frame 256 {
                    # "Slot 4: Big"
                    n330 = xnode "Motors"() -> ("Motor"=w761:T1)
                    n331 = Multiply(x="Slot 4: Big", y=-1) -> (x*y=w755:dbl)
                    n332 = xnode "Move a Fixed Distance"("Speed 1"=i8 -20, "Distance 1"=w755, "Motors"=w761) -> ("NXT/EV3"=w762:T2)  [unwired: 1 in]
                    n333 = call-poly <vilib>:"PolyWait.vi"("Time (1 sec)"=w759, "NXT/EV3"=w762) -> ("NXT/EV3"=w763:T2)  [unwired: 2 in]
                    n334 = xnode "Move a Fixed Distance"("Speed 1"=i8 20, "Distance 1"="Slot 4: Big", "Motors"=w761, "NXT/EV3"=w763) -> ()  [unwired: 1 out]
                  }
                  frame 512 {
                    # "Slot 4: Small"
                    n335 = xnode "Motors"() -> ("Motor"=w791:T1)
                    n336 = Multiply(x="Slot 4: Small", y=-1) -> (x*y=w786:dbl)
                    n337 = xnode "Move a Fixed Distance"("Speed 1"=i8 -20, "Distance 1"=w786, "Motors"=w791) -> ("NXT/EV3"=w792:T2)  [unwired: 1 in]
                    n338 = call-poly <vilib>:"PolyWait.vi"("Time (1 sec)"=w788, "NXT/EV3"=w792) -> ("NXT/EV3"=w793:T2)  [unwired: 2 in]
                    n339 = xnode "Move a Fixed Distance"("Speed 1"=i8 20, "Distance 1"="Slot 4: Small", "Motors"=w791, "NXT/EV3"=w793) -> ()  [unwired: 1 out]
                  }
                  frame 1024 {
                    # "Slot 5: Big"
                    n340 = xnode "Motors"() -> ("Motor"=w821:T1)
                    n341 = Multiply(x="Slot 5: Big", y=-1) -> (x*y=w816:dbl)
                    n342 = xnode "Move a Fixed Distance"("Speed 1"=i8 -20, "Distance 1"=w816, "Motors"=w821) -> ("NXT/EV3"=w822:T2)  [unwired: 1 in]
                    n343 = call-poly <vilib>:"PolyWait.vi"("Time (1 sec)"=w818, "NXT/EV3"=w822) -> ("NXT/EV3"=w823:T2)  [unwired: 2 in]
                    n344 = xnode "Move a Fixed Distance"("Speed 1"=i8 20, "Distance 1"="Slot 5: Big", "Motors"=w821, "NXT/EV3"=w823) -> ()  [unwired: 1 out]
                  }
                  frame 2048 {
                    # "Slot 5: Small"
                    n345 = xnode "Motors"() -> ("Motor"=w851:T1)
                    n346 = Multiply(x="Slot 5: Small", y=-1) -> (x*y=w847:dbl)
                    n347 = xnode "Move a Fixed Distance"("Speed 1"=i8 -20, "Distance 1"=w847, "Motors"=w851) -> ("NXT/EV3"=w852:T2)  [unwired: 1 in]
                    n348 = call-poly <vilib>:"PolyWait.vi"("Time (1 sec)"=w849, "NXT/EV3"=w852) -> ("NXT/EV3"=w853:T2)  [unwired: 2 in]
                    n349 = xnode "Move a Fixed Distance"("Speed 1"=i8 20, "Distance 1"="Slot 5: Small", "Motors"=w851, "NXT/EV3"=w853) -> ()  [unwired: 1 out]
                  }
                  frame 4096 {
                    # "Slot 6: Big"
                    n350 = xnode "Motors"() -> ("Motor"=w881:T1)
                    n351 = Multiply(x="Slot 6: Big", y=-1) -> (x*y=w877:dbl)
                    n352 = xnode "Move a Fixed Distance"("Speed 1"=i8 -20, "Distance 1"=w877, "Motors"=w881) -> ("NXT/EV3"=w882:T2)  [unwired: 1 in]
                    n353 = call-poly <vilib>:"PolyWait.vi"("Time (1 sec)"=w879, "NXT/EV3"=w882) -> ("NXT/EV3"=w883:T2)  [unwired: 2 in]
                    n354 = xnode "Move a Fixed Distance"("Speed 1"=i8 20, "Distance 1"="Slot 6: Big", "Motors"=w881, "NXT/EV3"=w883) -> ()  [unwired: 1 out]
                  }
                  frame 8192 {
                    # "Slot 6: Small"
                    n355 = xnode "Motors"() -> ("Motor"=w911:T1)
                    n356 = Multiply(x="Slot 6: Small", y=-1) -> (x*y=w906:dbl)
                    n357 = xnode "Move a Fixed Distance"("Speed 1"=i8 -20, "Distance 1"=w906, "Motors"=w911) -> ("NXT/EV3"=w912:T2)  [unwired: 1 in]
                    n358 = call-poly <vilib>:"PolyWait.vi"("Time (1 sec)"=w908, "NXT/EV3"=w912) -> ("NXT/EV3"=w913:T2)  [unwired: 2 in]
                    n359 = xnode "Move a Fixed Distance"("Speed 1"=i8 20, "Distance 1"="Slot 6: Small", "Motors"=w911, "NXT/EV3"=w913) -> ()  [unwired: 1 out]
                  }
                  frame 16384 {
                    # "Slot 7: Big"
                    n360 = xnode "Motors"() -> ("Motor"=w941:T1)
                    n361 = Multiply(x="Slot 7: Big", y=-1) -> (x*y=w937:dbl)
                    n362 = xnode "Move a Fixed Distance"("Speed 1"=i8 -20, "Distance 1"=w937, "Motors"=w941) -> ("NXT/EV3"=w942:T2)  [unwired: 1 in]
                    n363 = call-poly <vilib>:"PolyWait.vi"("Time (1 sec)"=w939, "NXT/EV3"=w942) -> ("NXT/EV3"=w943:T2)  [unwired: 2 in]
                    n364 = xnode "Move a Fixed Distance"("Speed 1"=i8 20, "Distance 1"="Slot 7: Big", "Motors"=w941, "NXT/EV3"=w943) -> ()  [unwired: 1 out]
                  }
                  frame 32768 {
                    # "Slot 7: Small"
                    n365 = xnode "Motors"() -> ("Motor"=w971:T1)
                    n366 = Multiply(x="Slot 7: Small", y=-1) -> (x*y=w966:dbl)
                    n367 = xnode "Move a Fixed Distance"("Speed 1"=i8 -20, "Distance 1"=w966, "Motors"=w971) -> ("NXT/EV3"=w972:T2)  [unwired: 1 in]
                    n368 = call-poly <vilib>:"PolyWait.vi"("Time (1 sec)"=w968, "NXT/EV3"=w972) -> ("NXT/EV3"=w973:T2)  [unwired: 2 in]
                    n369 = xnode "Move a Fixed Distance"("Speed 1"=i8 20, "Distance 1"="Slot 7: Small", "Motors"=w971, "NXT/EV3"=w973) -> ()  [unwired: 1 out]
                  }
                  frame 65536 {
                    # "Slot 8: Big"
                    n370 = xnode "Motors"() -> ("Motor"=w1001:T1)
                    n371 = Multiply(x="Slot 8: Big", y=-1) -> (x*y=w996:dbl)
                    n372 = xnode "Move a Fixed Distance"("Speed 1"=i8 -20, "Distance 1"=w996, "Motors"=w1001) -> ("NXT/EV3"=w1002:T2)  [unwired: 1 in]
                    n373 = call-poly <vilib>:"PolyWait.vi"("Time (1 sec)"=w998, "NXT/EV3"=w1002) -> ("NXT/EV3"=w1003:T2)  [unwired: 2 in]
                    n374 = xnode "Move a Fixed Distance"("Speed 1"=i8 20, "Distance 1"="Slot 8: Big", "Motors"=w1001, "NXT/EV3"=w1003) -> ()  [unwired: 1 out]
                  }
                  frame 131072 {
                    # "Slot 8: Small"
                    n375 = xnode "Motors"() -> ("Motor"=w1031:T1)
                    n376 = Multiply(x="Slot 8: Small", y=-1) -> (x*y=w1025:dbl)
                    n377 = xnode "Move a Fixed Distance"("Speed 1"=i8 -20, "Distance 1"=w1025, "Motors"=w1031) -> ("NXT/EV3"=w1032:T2)  [unwired: 1 in]
                    n378 = call-poly <vilib>:"PolyWait.vi"("Time (1 sec)"=w1028, "NXT/EV3"=w1032) -> ("NXT/EV3"=w1033:T2)  [unwired: 2 in]
                    n379 = xnode "Move a Fixed Distance"("Speed 1"=i8 20, "Distance 1"="Slot 8: Small", "Motors"=w1031, "NXT/EV3"=w1033) -> ()  [unwired: 1 out]
                  }
                }
              }
            }
            n380 = global read "all_done?.vi" "All Done?"() -> (w101:bool)
          }
        }
      }
    }
  }
